vi "delete module from engine.vi"(8 "error in":errorcluster, 10 "module ID":string, 11 "Standard Engine Configuration in":refnum<class "Standard Engine Configuration.lvclass">) -> (0 "error out":errorcluster, 3 "Standard Engine Configuration out":refnum<class "Standard Engine Configuration.lvclass">)   [LabVIEW 2013, in "Standard Engine Configuration.lvclass"]
doc: "Removes a module from the engine's list of modules to execute."
uses:
  Standard Engine Configuration.lvclass
  <vilib>/NI/Module Execution Interface/Engine Configuration/engine configuration.lvclass
  Standard Engine Configuration.lvclass/Standard Engine Configuration.ctl
  <vilib>/NI/Configuration Framework/serializable configuration/NISE_CEF_serializable configuration.lvclass/NISE_CEF_serializable configuration.ctl
  <vilib>/NI/Configuration Framework/serializable configuration/NISE_CEF_serializable configuration.lvclass
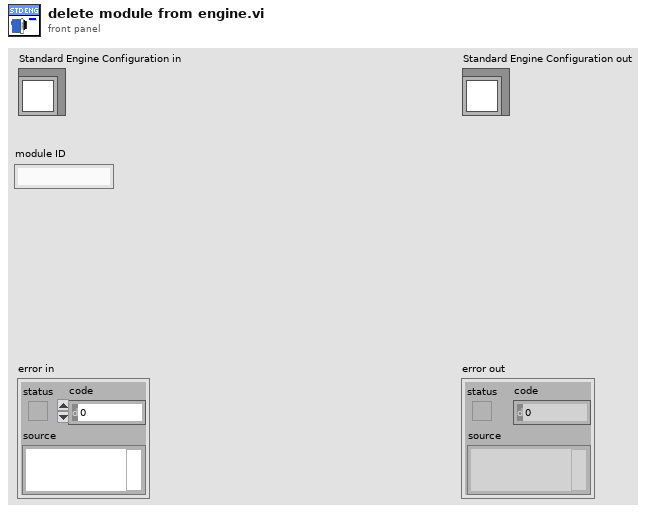
[diagram p1: front panel]
types:
  T1 = typedef "Standard Engine Configuration.lvclass/Module Specific Configuration.ctl" = cluster{"Module ID":string, "Module Decimation":T2, "error tag":string, "error responses":T3}
  T2 = typedef "Standard Engine Configuration.lvclass/Module Decimation.ctl" = cluster{"Decimation":u16, "Offset":u16, "sort order":i32, "async?":bool}
  T3 = typedef "Standard Engine Configuration.lvclass/error responses.ctl" = cluster{"unknown":T4, "trivial":T4, "critical":T4, "recoverable":T4}
  T4 = typedef "Standard Engine Configuration.lvclass/error options.ctl" = cluster{"clear":bool, "notify":bool, "remove module":bool, "abort engine":bool, "go to safe state":bool, "recover module":bool}
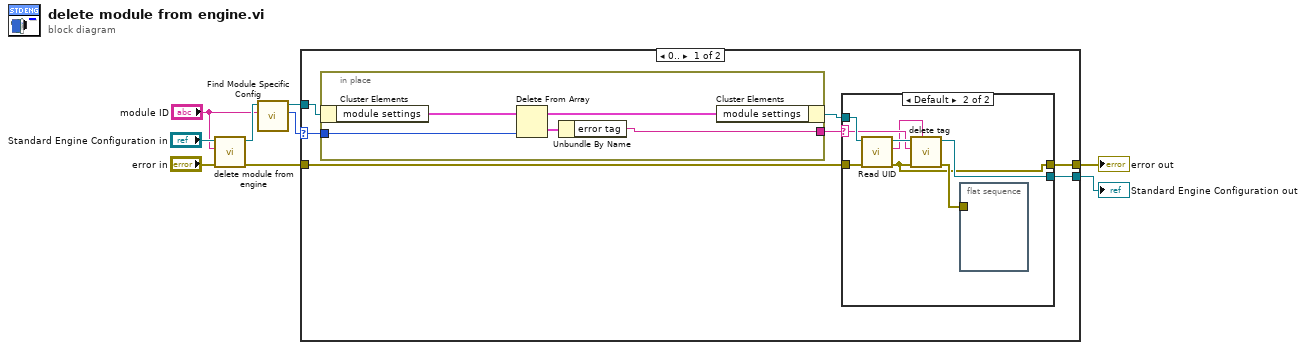
[diagram p0: block diagram]
diagram:
  n1 = call-parent "delete module from engine.vi"("error in"="error in", "module ID"="module ID", "engine configuration in"="Standard Engine Configuration in") -> ("error out"=w4:errorcluster, "engine configuration out"=w2:refnum<class "Standard Engine Configuration.lvclass">)  [unwired: 7 in]
  n2 = call "Find Module Specific Config.vi"("Module ID"="module ID", "Standard Engine Repo Data in"=w2) -> ("Index"=w6:i32, "Standard Engine Repo Data out"=w8:refnum<class "Standard Engine Configuration.lvclass">)  [unwired: 8 in]
  n3 = case shown="0.." w6 {
    selector: w6 -> [w15 _]
    tunnel: [w12 w33] -> w9
    tunnel: w8 -> [w16 w33]
    tunnel: w4 -> [w14 w32]
    tunnel: [w13 w32] -> w5
    frame 0.. {
      n4 = in-place {
        in-place-border: w15 -> [w29]
        in-place-border: [w27] -> w10
        n5 = in-place-cluster #1(w16) -> ("module settings"=w31:T1[])
        n6 = Delete From Array(array=w31, index=w29) -> (deleted portion=w28:T1, array with subset deleted=w30:T1[])  [unwired: 1 in]
        n7 = Unbundle By Name(w28) -> ("error tag"=w27:string)
        n8 = in-place-cluster #1("module settings"=w30) -> (w11:refnum<class "Standard Engine Configuration.lvclass">)
      }
      n9 = case shown="Default" w10 {
        selector: w10 -> [_ w20]
        tunnel: w14 -> [w18 w23]
        tunnel: [w18 w21] -> w13
        tunnel: [w17 w24] -> w12
        tunnel: w11 -> [w17 w26]
        frame "" {
        }
        frame Default {
          n10 = call <vilib>:"Read UID.vi"("error in"=w23, "configuration in"=w26) -> ("error out"=w21:errorcluster, "instance id"=w19:string, "configuration out"=w25:refnum<class "Standard Engine Configuration.lvclass">)  [unwired: 7 in]
          n11 = call <vilib>:"delete tag.vi"("owner ID"=w19, "error in"=w21, "tag name"=w20, "engine configuration in"=w25) -> ("error out"=w22:errorcluster, "engine configuration out"=w24:refnum<class "Standard Engine Configuration.lvclass">)  [unwired: 6 in]
          n12 = flat-sequence {
            tunnel: w22 -> [_]
            frame #0 {
            }
          }
        }
      }
    }
    frame ..-1 {
    }
  }
  "error out" <- w5
  "Standard Engine Configuration out" <- w9
